vi "shutdown process.vi"(8 "error in":errorcluster, 9 "timeout (500 ms)":u16=500, 11 "worker library":T2) -> (0 "error out":errorcluster, 2 "response fifos":T1)   [LabVIEW 2013, in "worker pool.lvlib"]
uses:
  worker pool.lvlib
  worker library reference.ctl
  worker comms.ctl
  worker commands.ctl
  request fifos.ctl
  recovery request.ctl
  <vilib>/NI/DCAF Module Framework/runtime/TBM module execution interface.lvclass
  <vilib>/NI/DCAF Module Framework/module configuration/TBM module configuration.lvclass
  rt fault.ctl
  <vilib>/NI/DCAF Module Framework/runtime/error classification.ctl
  response fifos.ctl
  recovery response.ctl
  <vilib>/NI/DCAF Execution Engine Interface/Engine Runtime/Fault.ctl
  <vilib>/NI/DCAF Execution Engine Interface/Engine Runtime/Engine Runtime Interface.lvclass
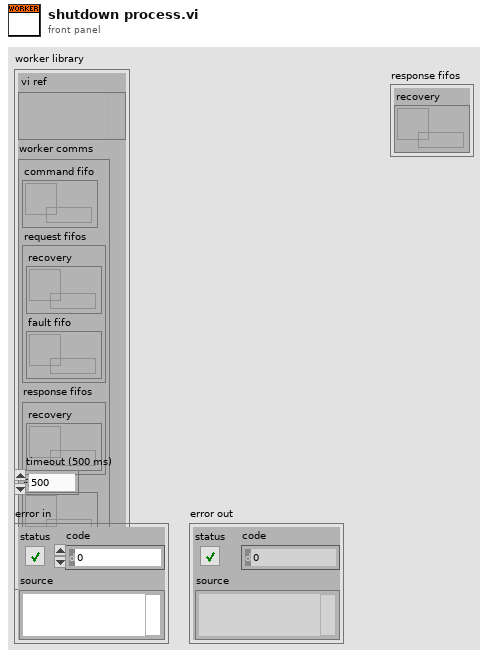
[diagram p1: front panel]
types:
  T1 = typedef "worker pool.lvlib/response fifos.ctl" = cluster{"recovery":refnum<k33>}
  T2 = typedef "worker pool.lvlib/worker library reference.ctl" = cluster{"vi ref":variant, "worker comms":T3, "worker count":i32}
  T3 = typedef "worker pool.lvlib/worker comms.ctl" = cluster{"command fifo":refnum<k33>, "request fifos":T4, "response fifos":T1, "fault list":refnum<data-value>}
  T4 = typedef "worker pool.lvlib/request fifos.ctl" = cluster{"recovery":refnum<k33>, "fault fifo":refnum<k33>}
  T5 = typedef "worker pool.lvlib/worker commands.ctl" = enum16{"shutdown", "recover module", "record fault"}
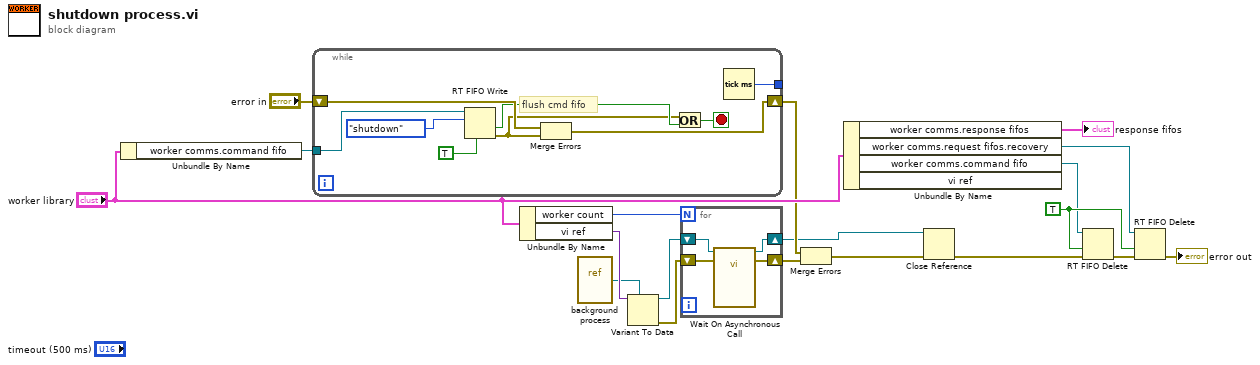
[diagram p0: block diagram]
diagram:
  w15 = TRUE ("force destroy? (F)")
  n1 = Unbundle By Name("worker library") -> ("worker comms.command fifo"=w19:refnum<k33>)
  n2 = while {
    tunnel: w19 -> [w28]
    shift-right: [w26] -> w8
    shift-left: "error in" -> [w25]
    tunnel: [w20] -> _
    stop <- w22 stop-if-true
    # "flush cmd fifo"
    n3 = RT FIFO Write(0:w28, 1:worker_commands."shutdown" ("element"), 5:TRUE ("overwrite on timeout (T)")) -> (10:w23:bool, 11:w21:errorcluster)  [unwired: 2 in, 2 out]
    n4 = Merge Errors(w25, w21) -> (w26:errorcluster)
    n5 = Or(x=w21, y=w23) -> (x .or. y?=w22:bool)
    n6 = Tick Count (ms)() -> (millisecond timer value=w20:u32)
  }
  n7 = Unbundle By Name("worker library") -> ("worker count"=w1:i32, "vi ref"=w9:variant)
  n8 = vi-ref "background process.vi"() -> (w7:refnum<vi>)
  n9 = Variant To Data(type=w7, Variant=w9) -> (data=w6:refnum<vi>, error out=w5:errorcluster)  [unwired: 1 in]
  n10 = for {
    N: w1 -> [_]
    shift-right: [w29] -> w2
    shift-left: w6 -> [w32]
    shift-right: [w30] -> w4
    shift-left: w5 -> [w31]
    n11 = call-by-ref "Wait On Asynchronous Call"(reference=w32, error in=w31) -> (reference out=w29:refnum<vi>, error out=w30:errorcluster)  [unwired: 12 in]
  }
  n12 = Merge Errors(w8, w4) -> (w3:errorcluster)
  n13 = Unbundle By Name("worker library") -> ("worker comms.response fifos"=→"response fifos":T1, "worker comms.request fifos.recovery"=w12:refnum<k33>, "worker comms.command fifo"=w13:refnum<k33>)  [unwired: 1 out]
  n14 = Close Reference(reference=w2, error in (no error)=w3) -> (error out=w16:errorcluster)
  n15 = RT FIFO Delete(0:w13, 2:w15, 3:w16) -> (11:w17:errorcluster)
  n16 = RT FIFO Delete(0:w12, 2:w15, 3:w17) -> (11:→"error out":errorcluster)
